vi "XNode Template Multiple.vi"(0 "failure in":T1 {"code" format="%.0x"}, 1 "Tags":string[](array[string]), 5 "Values":variant[](array[variant])) -> (4 "failure out":T1 {"code" format="%.0x"}, 8 "failed":bool)   [LabVIEW 2013, in "Write Exception Property.xnode"]
doc: "This VI is used to store data similar to a look up table, into a Variant data type. This VI is will set an attribute of the <b>Variant Repository In</b>, with the tags of <b>Tags</b>, value of <b>Values</b>, and then return the new <b>Varient Repository Out</b>. This VI will also return whether or not the new tags being written is replacing an old one or not, in the <b>Replaced?</b> boolean.\n\nThe tag name it self is optional and if one is not provided then the label name on the <b>Value</b> data will be used.\n\nOptionally the <b>Write Once?</b> boolean can be used. If true this will generate an error, if the tag that is trying to be written is already written. In this way the tag can only be written once without generating an error. By default this is set to false.\n\nTo read a single tag right click and choose Read Single Tag.\n\n-------------\nBrian Hoover (Hooovahh)\n\nProduct Name: Variant Repository\nPackage File Name: lava_lib_variant_repository\nPackage Version: 1.0.1.11\nMinimum LabVIEW Version: 11.0"
uses:
  Write Exception Property.xnode
  failure.ctl
  failure.lvlib
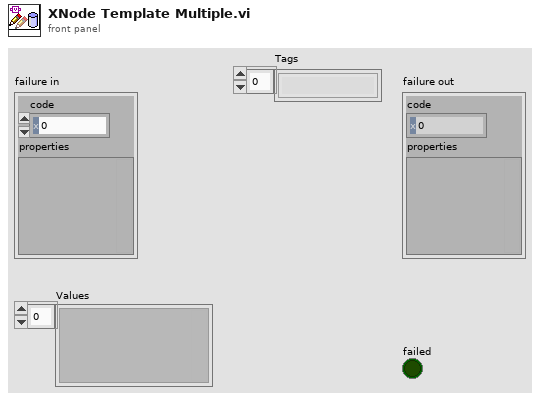
[diagram p1: front panel]
types:
  T1 = typedef "failure.lvlib/failure.ctl" = cluster{"code":i32, "properties":variant}
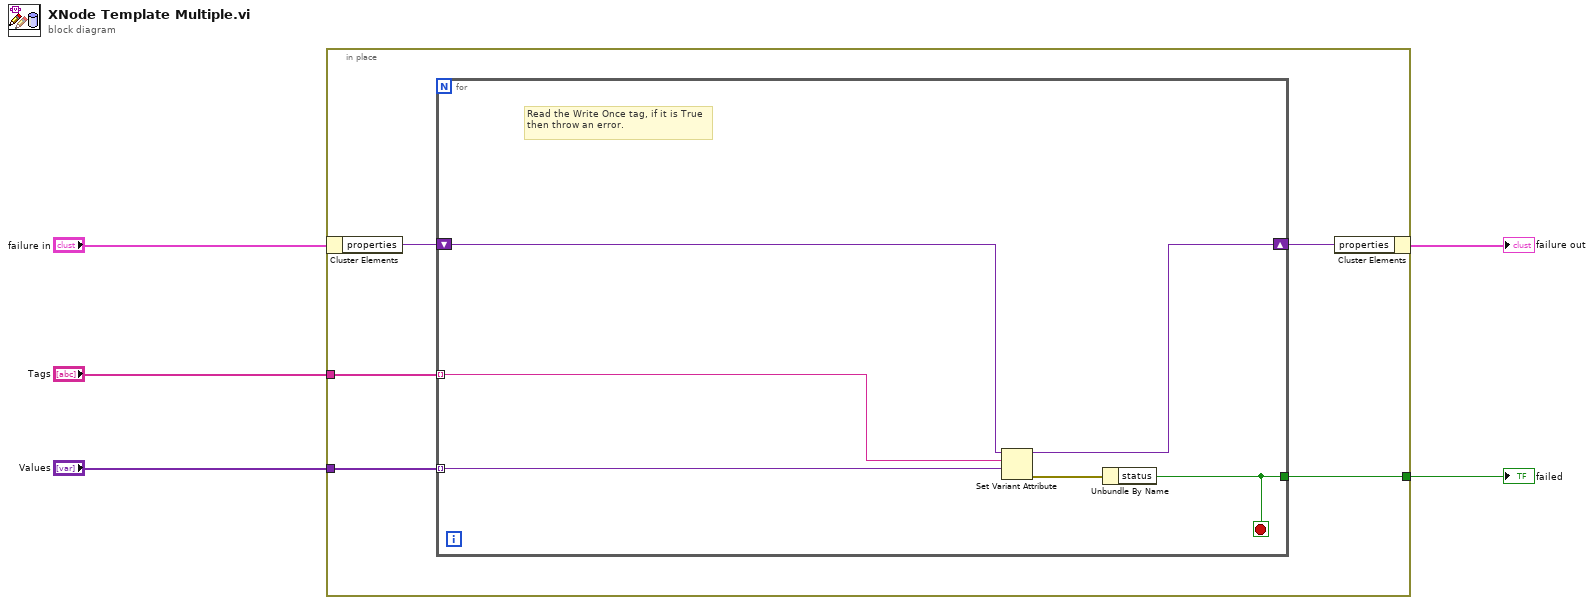
[diagram p0: block diagram]
diagram:
  n1 = in-place {
    in-place-border: "Tags" -> [w10]
    in-place-border: "Values" -> [w9]
    in-place-border: [w8] -> w3
    n2 = in-place-cluster #1("failure in") -> ("properties"=w7:variant)
    n3 = for {
      tunnel: [w15] -> w8
      tunnel: w9 -> [w16] mode=indexing
      tunnel: w10 -> [w12] mode=indexing
      shift-right: [w14] -> w6
      shift-left: w7 -> [w13]
      stop <- w15 stop-if-true
      # "Read the Write Once tag, if it is True then throw an error."
      n4 = Set Variant Attribute(Variant=w13, name=w12, value=w16) -> (Variant out=w14:variant, error out=w11:errorcluster)  [unwired: 1 in, 1 out]
      n5 = Unbundle By Name(w11) -> ("status"=w15:bool)
    }
    n6 = in-place-cluster #1("properties"=w6) -> (→"failure out":T1)
  }
  "failed" <- w3
